vi "WriteAOTFSettings.vi"(1 "error in (no error)":errorcluster) -> (0 "error out":errorcluster)   [LabVIEW 2009]
uses:
  AOTFSettings.ctt
  <vilib>/Utility/config.llb/NI_LVConfig.lvlib
panel:
  out "AOTF Setting":T1={"Laser 1 Output Channel"="5", "AOTF  1 Output Voltage"=2.0, "Laser 2 Output Channel"="6", "AOTF  2 Output Voltage"=4.0, "Laser 3 Output Channel"="1", "AOTF  3 Output Voltage"=8.0, "Pixel per Cycle"=0, "Time per Cycle  / ms"=10.0, "Laser 4 Output Channel"="1", "AOTF  4 Output Voltage"=0.0} {"AOTF  4 Output Voltage" format="%.2f"; "Time per Cycle  / ms" format="%#.3f"; "AOTF  3 Output Voltage" min=0.0 max=10.0 format="%.2f"; "AOTF  2 Output Voltage" min=0.0 max=10.0 format="%.2f"; "AOTF  1 Output Voltage" min=0.0 max=10.0 format="%.2f"}
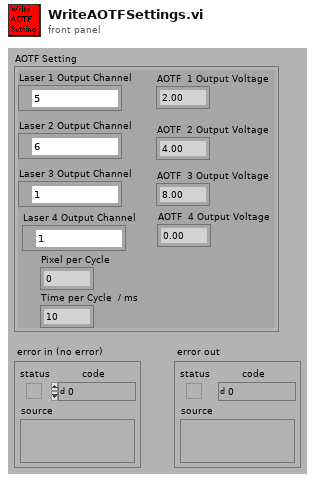
[diagram p1: front panel]
types:
  T1 = typedef "AOTFSettings.ctt" = cluster{"Laser 1 Output Channel":tag, "AOTF  1 Output Voltage":dbl, "Laser 2 Output Channel":tag, "AOTF  2 Output Voltage":dbl, "Laser 3 Output Channel":tag, "AOTF  3 Output Voltage":dbl, "Pixel per Cycle":u16, "Time per Cycle  / ms":dbl, "Laser 4 Output Channel":tag, "AOTF  4 Output Voltage":dbl}
  T2 = typedef "NI_LVConfig.lvlib/Config Data RefNum.ctl" = refnum<k1>
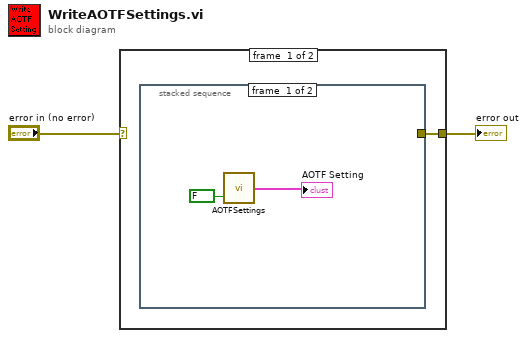
[diagram p0: block diagram]
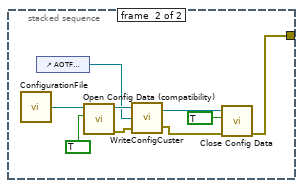
[diagram p2: hidden frame]
diagram:
  n1 = case shown="No Error" "error in (no error)" {
    selector: "error in (no error)" -> [_ w15]
    tunnel: [w3 w15] -> w1
    frame #0 {
      n2 = stacked-sequence {
        tunnel: [_ w7] -> w3
        frame #0 {
          n3 = call "AOTFSettings.vi"("Get/Set"=FALSE) -> ("AOTF Setting (Output)"=→"AOTF Setting":T1)  [unwired: 1 in]
        }
        frame #1 {
          n4 = call "ConfigurationFile.vi"() -> ("Configuration File (output)"=w10:path)  [unwired: 2 in]
          n5 = control-ref of="AOTF Setting"() -> (w6:refnum<vi>)
          n6 = call <vilib>:"Open Config Data (compatibility).vi"("create file if necessary (T)"=TRUE ("create file if necessary? (T)"), "configuration file path"=w10) -> ("error out"=w12:errorcluster, "refnum"=w13:T2)  [unwired: 7 in, 1 out]
          n7 = call "WriteConfigCuster.vi"("error in (no error)"=w12, "Ctrl Reference"=w6, "ConfigFile (input)"=w13) -> ("error out"=w8:errorcluster, "ConfigFile (output)"=w9:T2)
          n8 = call "Close Config Data.vi"("error in (no error)"=w8, "write configuration file? (T)"=TRUE ("write configuration file? (F)"), "refnum"=w9) -> ("error out"=w7:errorcluster)  [unwired: 8 in]
        }
      }
    }
    frame #1 {
    }
  }
  "error out" <- w1
